vi "set file meta.vi"(8 "error in (no error)":errorcluster, 11 "5785_2_x_200MHz in":refnum<class "5785_2_x_200MHz.lvclass">) -> (0 "error out":errorcluster, 3 "5785_2_x_200MHz out":refnum<class "5785_2_x_200MHz.lvclass">)   [LabVIEW 2021, in "5785_2_x_200MHz.lvclass"]
uses:
  5785_2_x_200MHz.lvclass
  5785_2_x_200MHz.lvclass/5785_2_x_200MHz.ctl
  pulse_tx_vis/device_mode.ctl
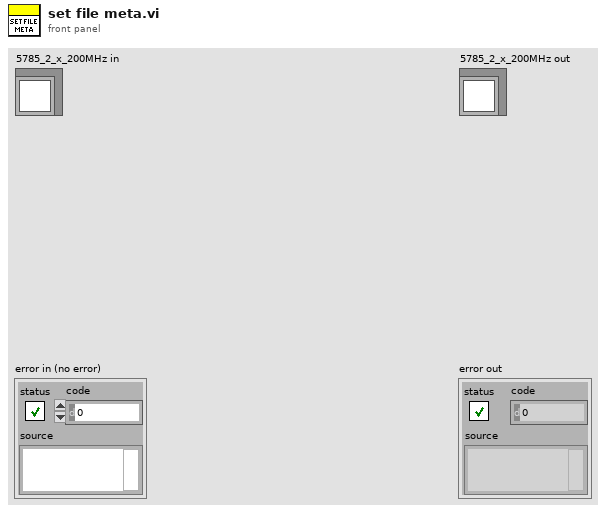
[diagram p1: front panel]
types:
  T1 = typedef "device_mode.ctl" = enum16{"USRP - 180MHz", "5785 - 2*180MHz", "5785 - 3.2GHz", "P2P - VST"}
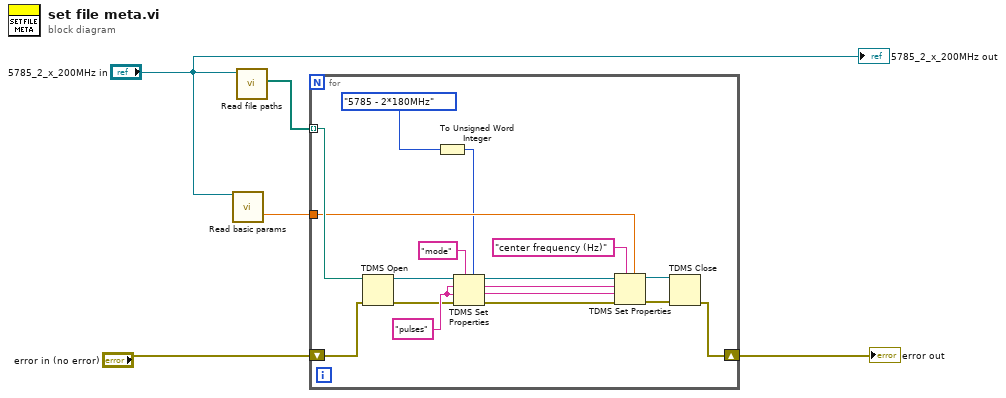
[diagram p0: block diagram]
diagram:
  n1 = call-dynamic "Read basic params.vi"("device_type in"="5785_2_x_200MHz in") -> ("center frequency (Hz)"=w1:dbl)  [unwired: 13 in, 5 out]
  n2 = call-dynamic "Read file paths.vi"("device_type in"="5785_2_x_200MHz in") -> ("file paths"=w5:path[])  [unwired: 8 in, 2 out]
  n3 = for {
    tunnel: w5 -> [w20] mode=indexing
    shift-right: [w8] -> w3
    shift-left: "error in (no error)" -> [w9]
    tunnel: w1 -> [w12]
    w22 = "pulses" ("channel name")
    n4 = TDMS Open(8:w9, 11:w20) -> (0:w19:errorcluster, 3:w21:refnum<k34>)  [unwired: 5 in]
    n5 = To Unsigned Word Integer(number=device_mode."5785 - 2*180MHz" ("Mode")) -> (unsigned 16bit integer=w6:u16)
    n6 = TDMS Set Properties(5:w6, 7:"mode", 8:w19, 9:w22, 10:w22, 11:w21) -> (0:w16:errorcluster, 1:w15:string, 2:w14:string, 3:w17:refnum<k34>)
    n7 = TDMS Set Properties(5:w12, 7:"center frequency (Hz)", 8:w16, 9:w15, 10:w14, 11:w17) -> (0:w10:errorcluster, 3:w11:refnum<k34>)  [unwired: 2 out]
    n8 = TDMS Close(8:w10, 11:w11) -> (0:w8:errorcluster)  [unwired: 1 out]
  }
  "error out" <- w3
  "5785_2_x_200MHz out" <- "5785_2_x_200MHz in"
